vi "SetParameter.vi"(8 "error in (no error)":errorcluster, 10 "InClusTiming":T1={"Pixelclock"=24, "Exposure"=46.39115, "ExposureTimeBase"=2, "Framerate"=14.99615, "TriggerMode"=0} {"TriggerMode" items=["Auto", "Software", "External sequence start ", "External exposure control"]; "ExposureTimeBase" items=["nanoseconds", "microseconds", "milliseconds"]; "Pixelclock" min=1 max=150 step=1 scale=0.05915..150.0; "Framerate" min=0.05915 max=2000.0 step=1.0 scale=0.05915..100.0 scale format="%#.3g"; "Exposure" min=0.001 max=400.0 step=0.001 scale=0.05915..400.0 scale format="%#.3g"}, 11 "HAMAMATSU_DCAMAPI in":refnum<class "HAMAMATSU_DCAMAPI.lvclass">) -> (0 "error out":errorcluster, 3 "HAMAMATSU_DCAMAPI out":refnum<class "HAMAMATSU_DCAMAPI.lvclass">)   [LabVIEW 2020, in "HAMAMATSU_DCAMAPI.lvclass"]
uses:
  HAMAMATSU_DCAMAPI.lvclass
  Image Acquisition Class/Camera.lvclass
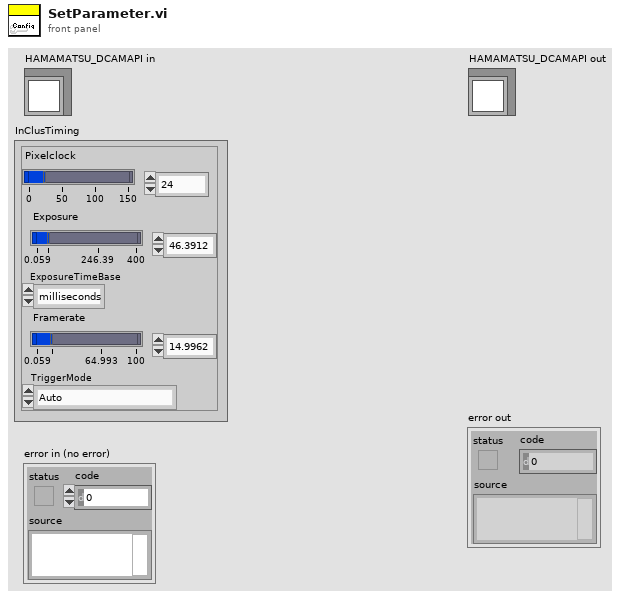
[diagram p1: front panel]
types:
  T1 = cluster{"Pixelclock":i32, "Exposure":dbl, "ExposureTimeBase":u16, "Framerate":dbl, "TriggerMode":u16}
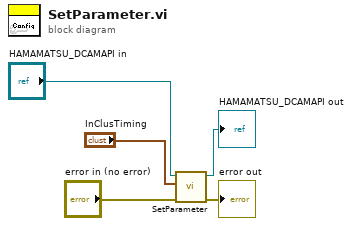
[diagram p0: block diagram]
diagram:
  n1 = call-parent "SetParameter.vi"("error in (no error)"="error in (no error)", "InClusTiming"="InClusTiming", "Camera in"="HAMAMATSU_DCAMAPI in") -> ("error out"=→"error out":errorcluster, "Camera out"=→"HAMAMATSU_DCAMAPI out":refnum<class "HAMAMATSU_DCAMAPI.lvclass">)  [unwired: 7 in]
